vi "HEXMOVE.vi"() -> ()   [LabVIEW 2011]
panel:
  in  "OK Button 12":bool
  in  "OK Button 10":bool
  in  "OK Button 9":bool
  in  "OK Button 8":bool
  in  "OK Button 6":bool
  in  "OK Button 4":bool
  in  "OK Button 13":bool
  in  "OK Button 11":bool
  in  "OK Button 5":bool
  in  "OK Button 3":bool
  in  "OK Button 2":bool
  in  "OK Button 7":bool
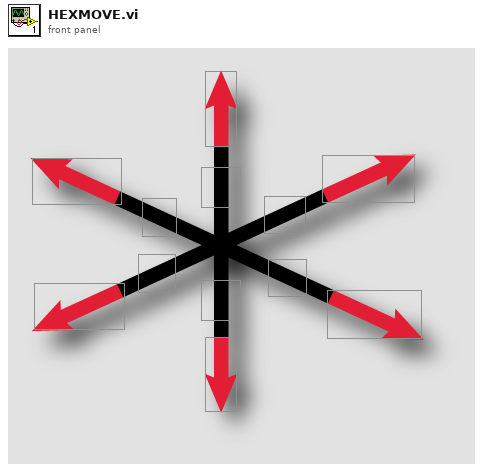
[diagram p1: front panel]
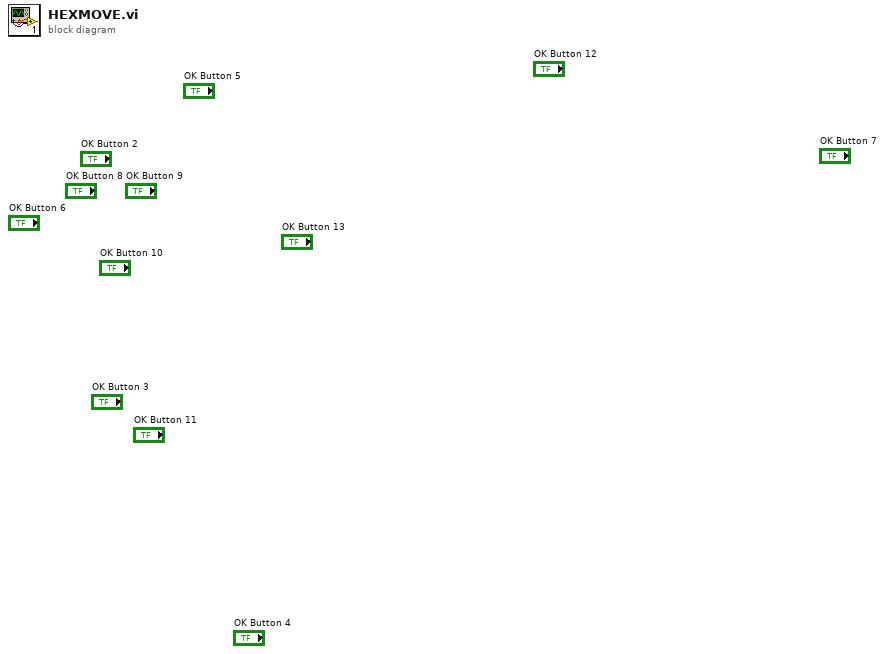
[diagram p0: block diagram]
diagram:
